vi "NI-DCPower Specific Logic.vi"(7 "connections":T1[](array[typedef]), 8 "error in":errorcluster, 9 "channel list":string, 10 "instrument handle":refnum<k15>, 11 "Measurement Configuration":T4={"pin_names"=[], "voltage_level"=6.0, "voltage_level_range"=6.0, "current_limit"=0.01, "current_limit_range"=0.01, "source_delay"=0.0}) -> (0 "error out":errorcluster, 2 "instrument handle out":refnum<k15>, 3 "Measurement Results":T3)   [LabVIEW 2021, in "NIDCPowerSourceDCVoltage.lvlib"]
uses:
  NIDCPowerSourceDCVoltage.lvlib
  Measurement Configuration.ctl
  Measurement Results.ctl
  <vilib>/Plug-In SDKs/Sessions/niDCPower/Connection with Session.ctl
  <vilib>/Plug-In SDKs/Clients/Session Management V1/Session Reservation/Connection.ctl
  <instrlib>/niDCPower/nidcpower.llb/niDCPower Source Mode.ctl
  <instrlib>/niDCPower/nidcpower.llb/niDCPower Output Function.ctl
  <instrlib>/niDCPower/nidcpower.llb/niDCPower Wait For Event - Event.ctl
  <vilib>/Plug-In SDKs/Clients/Session Management V1/Session Reservation/Session Reservation.lvclass
  <vilib>/Plug-In SDKs/Sessions/niDCPower/NI Session Management niDCPower.lvlib
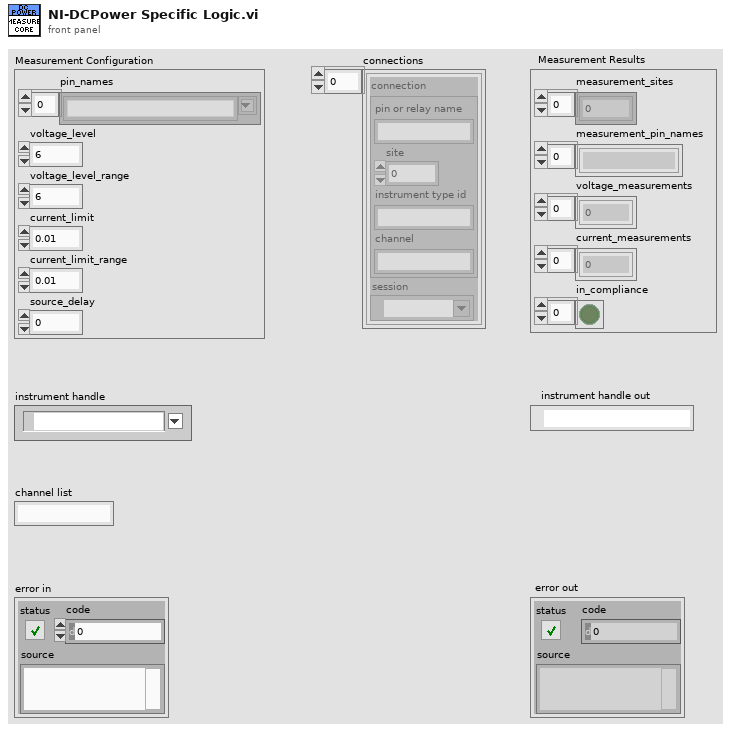
[diagram p1: front panel]
types:
  T1 = typedef "NI Session Management niDCPower.lvlib/Connection with Session.ctl" = cluster{"connection":T2, "session":refnum<k15>}
  T2 = typedef "NI Session Management V1 Client.lvlib/Session Reservation.lvclass/Connection.ctl" = cluster{"pin or relay name":string, "site":i32, "instrument type id":string, "channel":string}
  T3 = typedef "NIDCPowerSourceDCVoltage.lvlib/Measurement Results.ctl" = cluster{"measurement_sites":i32[], "measurement_pin_names":string[], "voltage_measurements":dbl[], "current_measurements":dbl[], "in_compliance":bool[]}
  T4 = typedef "NIDCPowerSourceDCVoltage.lvlib/Measurement Configuration.ctl" = cluster{"pin_names":string[], "voltage_level":dbl, "voltage_level_range":dbl, "current_limit":dbl, "current_limit_range":dbl, "source_delay":dbl}
  T5 = typedef "niDCPower Wait For Event - Event.ctl" = i32
  T6 = typedef "niDCPower Output Function.ctl" = i32
  T7 = typedef "niDCPower Source Mode.ctl" = i32
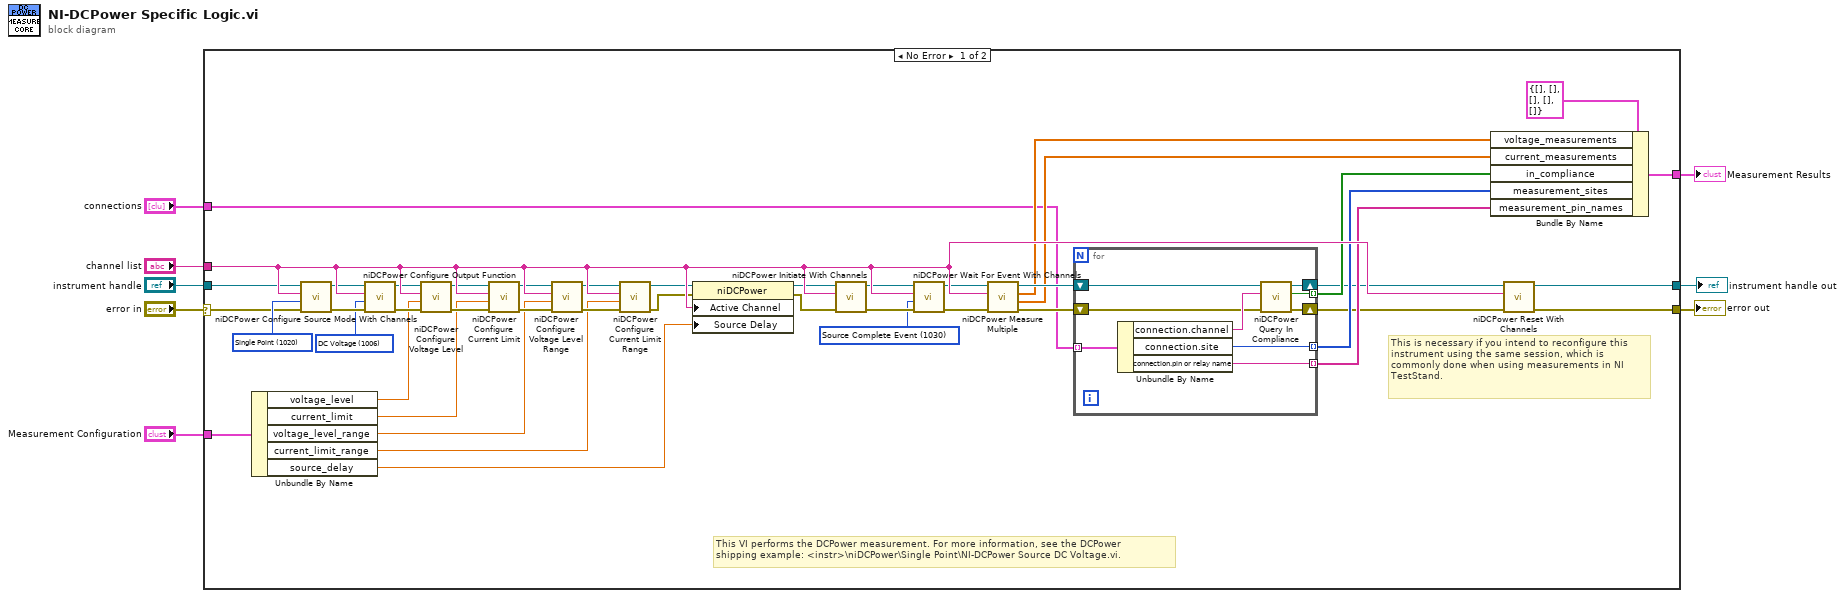
[diagram p0: block diagram]
diagram:
  n1 = case shown="No Error" "error in" {
    selector: "error in" -> [w13 w62]
    tunnel: "Measurement Configuration" -> [w28 _]
    tunnel: [w23 _] -> w7
    tunnel: [w11 w62] -> w6
    tunnel: "instrument handle" -> [w14 w63]
    tunnel: [w9 w63] -> w4
    tunnel: "channel list" -> [w52 _]
    tunnel: "connections" -> [w12 _]
    frame No Error {
      w29 = T5 1030 items=["Source Complete Event"=1030, "Measure Complete Event"=1031, "Sequence Iteration Complete Event"=1032, "Sequence Engine Done Event"=1033, "Pulse Complete Event"=1051, "Ready For Pulse Trigger Event"=1052] ("event")
      w32 = T6 1006 items=["DC Voltage"=1006, "DC Current"=1007, "Pulse Voltage"=1049, "Pulse Current"=1050] ("output function")
      w33 = T7 1020 items=["Single Point"=1020, "Sequence"=1021] ("source mode")
      # "This is necessary if you intend to reconfigure this instrument using the same session, which is commonly done when using measurements in NI TestStand."
      # "This VI performs the DCPower measurement. For more information, see the DCPower\nshipping example: <instr>\\niDCPower\\Single Point\\NI-DCPower Source DC Voltage.vi."
      n2 = Unbundle By Name(w28) -> ("voltage_level"=w31:dbl, "current_limit"=w30:dbl, "voltage_level_range"=w27:dbl, "current_limit_range"=w26:dbl, "source_delay"=w25:dbl)
      n3 = call <instrlib>:"niDCPower Configure Source Mode With Channels.vi"("error in (no error)"=w13, "source mode"=w33, "channel name"=w52, "instrument handle"=w14) -> ("error out"=w49:errorcluster, "instrument handle out"=w48:refnum<k15>)  [unwired: 6 in]
      n4 = call <instrlib>:"niDCPower Configure Output Function.vi"("error in (no error)"=w49, "output function"=w32, "channel name"=w52, "instrument handle"=w48) -> ("error out"=w34:errorcluster, "instrument handle out"=w35:refnum<k15>)  [unwired: 6 out]
      n5 = call <instrlib>:"niDCPower Configure Voltage Level.vi"("error in (no error)"=w34, "voltage level"=w31, "channel name"=w52, "instrument handle"=w35) -> ("error out"=w50:errorcluster, "instrument handle out"=w51:refnum<k15>)  [unwired: 6 out]
      n6 = call <instrlib>:"niDCPower Configure Current Limit.vi"("error in (no error)"=w50, "current limit"=w30, "channel name"=w52, "instrument handle"=w51) -> ("error out"=w47:errorcluster, "instrument handle out"=w46:refnum<k15>)  [unwired: 1 in, 5 out]
      n7 = call <instrlib>:"niDCPower Configure Voltage Level Range.vi"("error in (no error)"=w47, "voltage level range"=w27, "channel name"=w52, "instrument handle"=w46) -> ("error out"=w45:errorcluster, "instrument handle out"=w44:refnum<k15>)  [unwired: 6 out]
      n8 = call <instrlib>:"niDCPower Configure Current Limit Range.vi"("error in (no error)"=w45, "current limit range"=w26, "channel name"=w52, "instrument handle"=w44) -> ("error out"=w40:errorcluster, "instrument handle out"=w43:refnum<k15>)  [unwired: 6 out]
      n9 = property class="niDCPower"(reference=w43, error in=w40, "Active Channel"=w52, "Source Delay"=w25) -> (reference out=w42:refnum<k15>, error out=w41:errorcluster)
      n10 = call <instrlib>:"niDCPower Initiate With Channels.vi"("error in (no error)"=w41, "channel name"=w52, "instrument handle"=w42) -> ("error out"=w37:errorcluster, "instrument handle out"=w39:refnum<k15>)  [unwired: 7 in]
      n11 = call <instrlib>:"niDCPower Wait For Event With Channels.vi"("error in (no error)"=w37, "event"=w29, "channel name"=w52, "instrument handle"=w39) -> ("error out"=w36:errorcluster, "instrument handle out"=w38:refnum<k15>)  [unwired: 6 in]
      n12 = call <instrlib>:"niDCPower Measure Multiple.vi"("error in (no error)"=w36, "channel name"=w52, "instrument handle"=w38) -> ("error out"=w21:errorcluster, "current measurements"=w19:dbl[], "voltage measurements"=w20:dbl[], "instrument handle out"=w22:refnum<k15>)  [unwired: 5 out]
      n13 = for {
        tunnel: w12 -> [w61] mode=indexing
        tunnel: [w60] -> w17 mode=indexing
        tunnel: [w59] -> w16 mode=indexing
        shift-right: [w56] -> w10
        shift-left: w22 -> [w57]
        shift-right: [w54] -> w15
        shift-left: w21 -> [w55]
        tunnel: [w53] -> w18 mode=indexing
        n14 = Unbundle By Name(w61) -> ("connection.channel"=w58:string, "connection.site"=w60:i32, "connection.pin or relay name"=w59:string)
        n15 = call <instrlib>:"niDCPower Query In Compliance.vi"("error in (no error)"=w55, "channel name"=w58, "instrument handle"=w57) -> ("error out"=w54:errorcluster, "in compliance?"=w53:bool, "instrument handle out"=w56:refnum<k15>)  [unwired: 6 out]
      }
      n16 = Bundle By Name(cluster=T3 {"measurement_sites"=[], "measurement_pin_names"=[], "voltage_measurements"=[], "current_measurements"=[], "in_compliance"=[]} ("Measurement Results"), "voltage_measurements"=w20, "current_measurements"=w19, "in_compliance"=w18, "measurement_sites"=w17, "measurement_pin_names"=w16) -> (w23:T3)
      n17 = call <instrlib>:"niDCPower Reset With Channels.vi"("error in (no error)"=w15, "channel name"=w52, "instrument handle"=w10) -> ("error out"=w11:errorcluster, "instrument handle out"=w9:refnum<k15>)  [unwired: 7 in]
    }
    frame Error {
    }
  }
  "Measurement Results" <- w7
  "error out" <- w6
  "instrument handle out" <- w4
